vi "1. vision影像擷取.vi"() -> ()   [LabVIEW 2017]
uses:
  <vilib>/vision/driver/NI_Vision_Acquisition_Software.lvlib
panel:
  out "顯示錯誤":errorcluster
  out "Camera Information Array":T1(array[cluster]) {"BusType" format="%x"; "SerialNumberLow" format="%.0x"; "SerialNumberHigh" format="%.0x"}
  out "影像":T2(plugin-control)
  in  "stop":bool
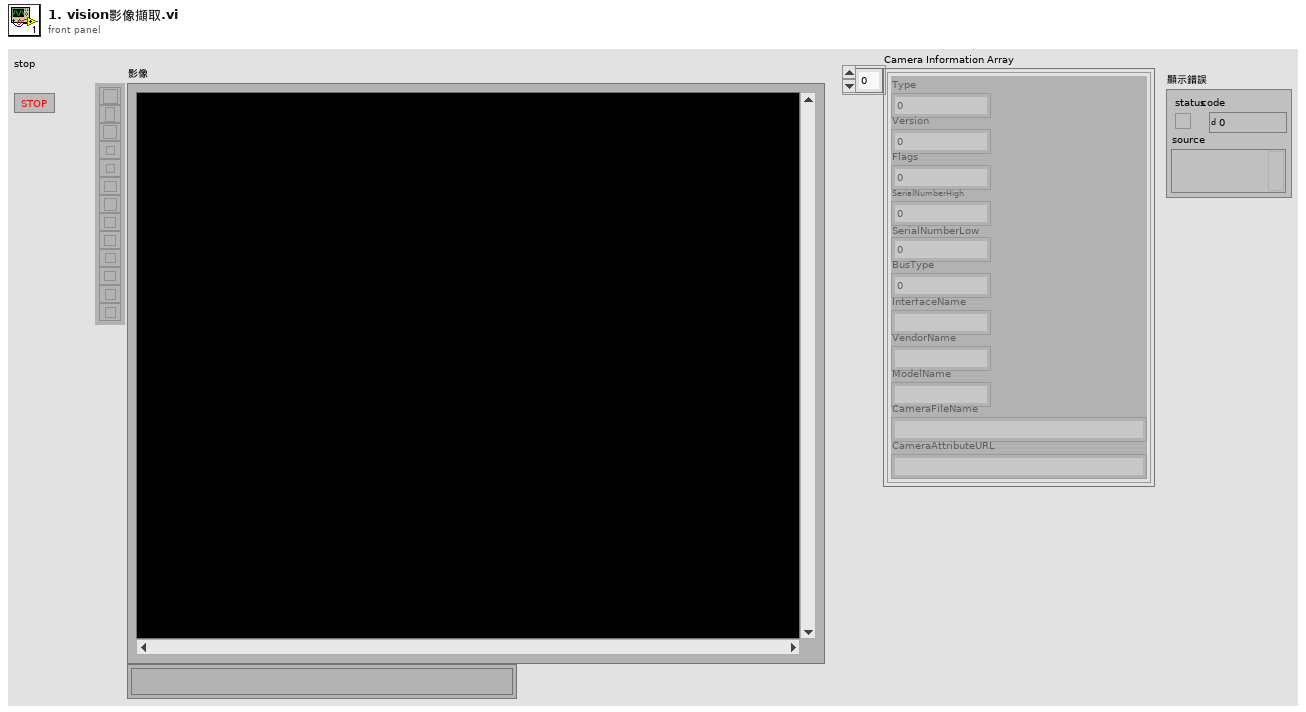
[diagram p1: front panel]
types:
  T1 = cluster{"Type":u32, "Version":u32, "Flags":u32, "SerialNumberHigh":u32, "SerialNumberLow":u32, "BusType":u32, "InterfaceName":string, "VendorName":string, "ModelName":string, "CameraFileName":string, "CameraAttributeURL":string}[]
  T2 = typedef "IMAQ Image.ctl" = refnum<image>
  T3 = typedef "Image Type" = u32
  T4 = cluster{"Type":u32, "Version":u32, "Flags":u32, "SerialNumberHigh":u32, "SerialNumberLow":u32, "BusType":u32, "InterfaceName":string, "VendorName":string, "ModelName":string, "CameraFileName":string, "CameraAttributeURL":string}
  T5 = typedef "IMAQdx.ctl" = refnum<k21>
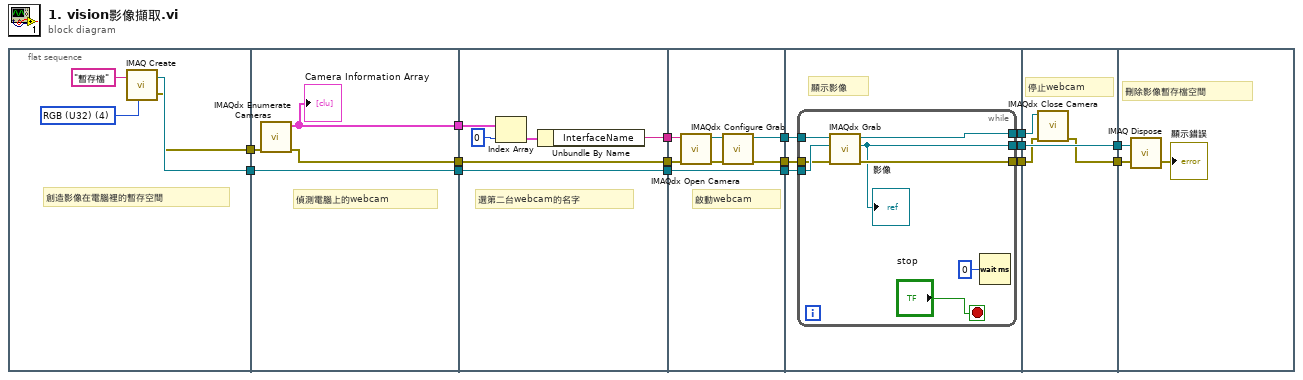
[diagram p0: block diagram]
diagram:
  n1 = flat-sequence {
    tunnel: [w18] -> w7
    tunnel: [w17] -> w6
    tunnel: [w24] -> w16
    tunnel: [w23] -> w8
    tunnel: w7 -> [w23]
    tunnel: w6 -> [w22]
    tunnel: [w21] -> w4
    tunnel: w16 -> [w28]
    tunnel: [w27] -> w15
    tunnel: [w26] -> w9
    tunnel: w8 -> [w26]
    tunnel: [w25] -> w5
    tunnel: w4 -> [w25]
    tunnel: w15 -> [w36]
    tunnel: [w35] -> w14
    tunnel: [w34] -> w10
    tunnel: w9 -> [w34]
    tunnel: w5 -> [w33]
    tunnel: [w31] -> w3
    tunnel: w14 -> [w43]
    tunnel: [w42] -> w13
    tunnel: [w41] -> w11
    tunnel: w10 -> [w40]
    tunnel: w3 -> [w39]
    tunnel: [w38] -> w2
    tunnel: w13 -> [w55]
    tunnel: [w54] -> w12
    tunnel: w11 -> [w54]
    tunnel: w2 -> [w53]
    tunnel: [w52] -> w1
    tunnel: w12 -> [w58]
    tunnel: w1 -> [w57]
    frame #0 {
      w20 = T3 4 items=["Grayscale (U8)", "Grayscale (I16)", "Grayscale (SGL)", "Complex (CSG)", "RGB (U32)", "HSL (U32)", "RGB (U64)", "Grayscale (U16)"] ("Image Type")
      # "創造影像在電腦裡的暫存空間"
      n2 = call "IMAQ Create"("Image Name"="暫存檔", "Image Type"=w20) -> ("New Image"=w18:T2, "error out"=w17:errorcluster)  [unwired: 3 in]
    }
    frame #1 {
      # "偵測電腦上的webcam"
      n3 = call <vilib>:"IMAQdx Enumerate Cameras.vi"("error in"=w22) -> ("error out"=w21:errorcluster, "Camera Information Array"=w24:T1)  [unwired: 9 in]
      "Camera Information Array" <- w24
    }
    frame #2 {
      # "選第二台webcam的名字"
      n4 = Index Array(array=w28, index=0) -> (element=w29:T4)
      n5 = Unbundle By Name(w29) -> ("InterfaceName"=w27:string)
    }
    frame #3 {
      # "啟動webcam"
      n6 = call <vilib>:"IMAQdx Open Camera.vi"("error in"=w33, "Session In"=w36) -> ("error out"=w32:errorcluster, "Session Out"=w37:T5)  [unwired: 8 in]
      n7 = call <vilib>:"IMAQdx Configure Grab.vi"("error in"=w32, "Session In"=w37) -> ("error out"=w31:errorcluster, "Session Out"=w35:T5)  [unwired: 8 in]
    }
    frame #4 {
      # "顯示影像"
      n8 = while {
        tunnel: [w50] -> w42
        tunnel: [w45] -> w41
        tunnel: w43 -> [w49]
        tunnel: w40 -> [w48]
        tunnel: w39 -> [w47]
        tunnel: [w46] -> w38
        stop <- "stop" stop-if-true
        n9 = call <vilib>:"IMAQdx Grab.vi"("error in"=w47, "Image In"=w48, "Session In"=w49) -> ("error out"=w46:errorcluster, "Image Out"=w45:T2, "Session Out"=w50:T5)  [unwired: 5 in, 1 out]
        "影像" <- w45
        n10 = Wait (ms)(milliseconds to wait=u32 0) -> ()  [unwired: 1 out]
      }
    }
    frame #5 {
      # "停止webcam"
      n11 = call <vilib>:"IMAQdx Close Camera.vi"("error in"=w53, "Session In"=w55) -> ("error out"=w52:errorcluster)  [unwired: 9 in]
    }
    frame #6 {
      # "刪除影像暫存檔空間"
      n12 = call "IMAQ Dispose"("Image"=w58, "error in (no error)"=w57) -> ("error out"=→"顯示錯誤":errorcluster)  [unwired: 4 in]
    }
  }
